vi "Get Node Label.vi"(11 "Node in":variant) -> (2 "Node Label":string, 3 "Node out":variant)   [LabVIEW 2021, in "GraphLib.lvlib" / "Abstract Graph.lvclass"]
uses:
  Abstract Graph.lvclass
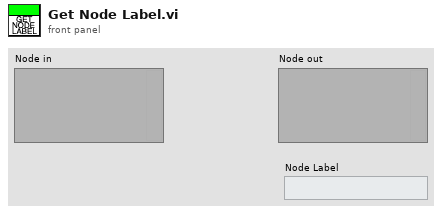
[diagram p1: front panel]
types:
  T1 = typedef "Type Descriptor Enumeration__ogtk.ctl" = enum8{"<Null>", "I8", "I16", "I32", "I64", "U8", "U16", "U32", "U64", "SGL", "DBL", "EXT", "CSG", "CDB", "CXT", "0x0F", "0x10", "0x11", "0x12", "0x13", "0x14", "Enum U8", "Enum U16", "Enum U32", "Enum U64", "SGL PQ", "DBL PQ", "EXT PQ", "CSG PQ", "CDB PQ", "CXT PQ", "0x1F", "0x20", "Boolean", "0x22", "0x23", "0x24", "0x25", "0x26", "0x27", "0x28", "0x29", "0x2A", "0x2B", "0x2C", "0x2D", "0x2E", "0x2F", "String", "0x31", "Path", "Pict", "0x34", "0x35", "0x36", "DAQ", "0x38", "0x39", "0x3A", "0x3B", "0x3C", "0x3D", "0x3E", "0x3F", "Array", "0x41", "0x42", "0x43", "0x44", "0x45", "0x46", "0x47", "0x48", "0x49", "0x4A", "0x4B", "0x4C", "0x4D", "0x4E", "0x4F", "Cluster", "0x51", "0x52", "Variant", "Waveform", "0x55", "0x56", "0x57", "0x58", "0x59", "0x5A", "0x5B", "0x5C", "0x5D", "0x5E", "Fixed Point", "0x60", "0x61", "0x62", "0x63", "0x64", "0x65", "0x66", "0x67", "0x68", "0x69", "0x6A", "0x6B", "0x6C", "0x6D", "0x6E", "0x6F", "Refnum", "0x71", "0x72", "Set Collection", "Map Collection"}
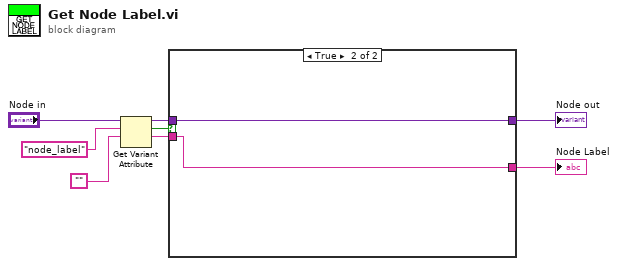
[diagram p0: block diagram]
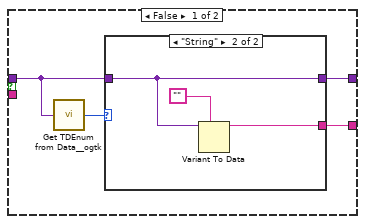
[diagram p2: hidden frame]
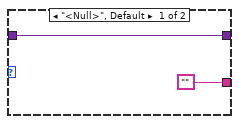
[diagram p3: hidden frame]
diagram:
  n1 = Get Variant Attribute(Variant="Node in", name="node_label", default value (empty Variant)="") -> (duplicate Variant=w4:variant, found=w5:bool, value=w1:string)  [unwired: 1 in, 1 out]
  n2 = case shown="True" w5 {
    tunnel: w4 -> [w11 w19]
    tunnel: [w10 w18] -> w3
    tunnel: [w9 w19] -> w2
    tunnel: w1 -> [_ w18]
    frame False {
      n3 = call <userlib>:"Get TDEnum from Data__ogtk.vi"("Data"=w11) -> ("Type Descriptor Enumeration"=w12:T1)  [unwired: 4 in]
      n4 = case shown="\"String\"" w12 {
        tunnel: w11 -> [w14 w15]
        tunnel: ["" w16] -> w10
        tunnel: [w14 w15] -> w9
        frame "<Null>", Default {
        }
        frame "String" {
          n5 = Variant To Data(type="", Variant=w15) -> (data=w16:string)  [unwired: 1 in, 1 out]
        }
      }
    }
    frame True {
    }
  }
  "Node out" <- w2
  "Node Label" <- w3
